vi "disdrometer_weathericon.vi"(0 "Weather Status":string, 5 "Time (seconds, GMT)":dbl, 7 "Offset (hours)":dbl, 9 "Begin Daylight (hours)":dbl=8.0, 11 "End Daylight (hours)":dbl=20.0) -> (6 "String":string, 10 "Icon":picture)   [LabVIEW 2018]
doc: "Accepts a SYNOP Tab.4680 weather code (e.g. \"R-\", \"R \", \"R+\", etc.) and returns a string description and the filepath to an associated icon.\n\nTime parameters can be optionally included to vary the icon based on a day/night cycle."
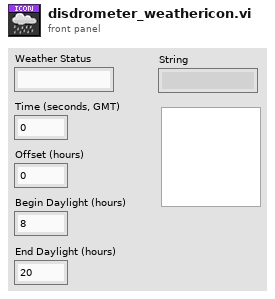
[diagram p1: front panel]
types:
  T1 = typedef "imagedata.ctl" = cluster{"image type":i32, "image depth":i32, "image":u8[], "mask":u8[], "colors":u32[], "Rectangle":cluster{"left":i16, "top":i16, "right":i16, "bottom":i16}}
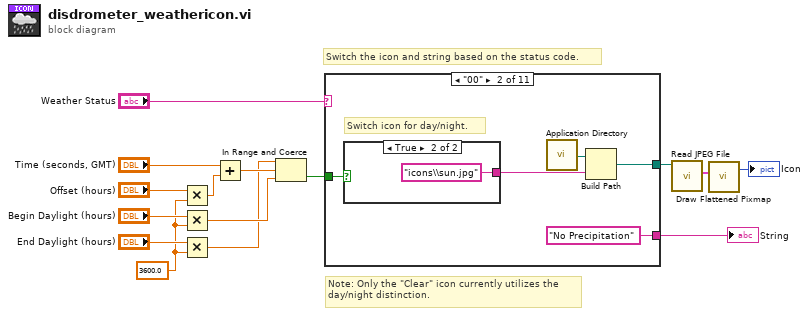
[diagram p0: block diagram]
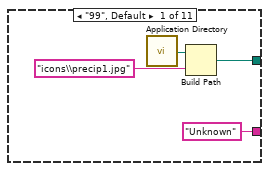
[diagram p2: hidden frame]
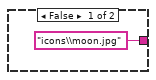
[diagram p3: hidden frame]
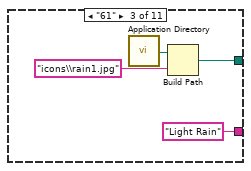
[diagram p4: hidden frame]
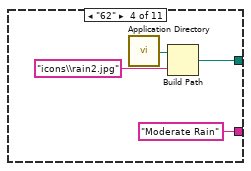
[diagram p5: hidden frame]
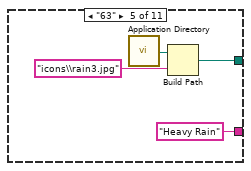
[diagram p6: hidden frame]
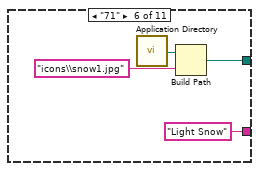
[diagram p7: hidden frame]
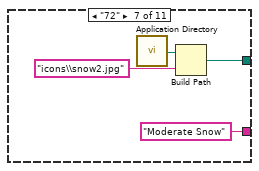
[diagram p8: hidden frame]
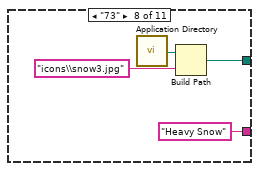
[diagram p9: hidden frame]
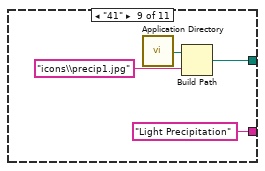
[diagram p10: hidden frame]
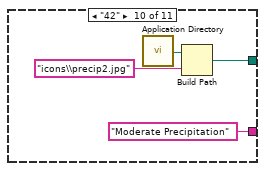
[diagram p11: hidden frame]
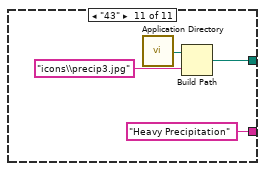
[diagram p12: hidden frame]
diagram:
  w6 = 3600.0 ("y")
  # "Switch the icon and string based on the status code."
  # "Note: Only the \"Clear\" icon currently utilizes the\nday/night distinction."
  n1 = Multiply(x="Offset (hours)", y=w6) -> (x*y=w10:dbl)
  n2 = Multiply(x="Begin Daylight (hours)", y=w6) -> (x*y=w5:dbl)
  n3 = Multiply(x="End Daylight (hours)", y=w6) -> (x*y=w4:dbl)
  n4 = Add(x="Time (seconds, GMT)", y=w10) -> (x+y=w8:dbl)
  n5 = In Range and Coerce(upper limit=w4, x=w8, lower limit=w5) -> (In Range?=w15:bool)  [unwired: 1 out]
  n6 = case shown="\"00\"" "Weather Status" {
    tunnel: ["Unknown" "No Precipitation" "Light Rain" "Moderate Rain" "Heavy Rain" "Light Snow" "Moderate Snow" "Heavy Snow" "Light Precipitation" "Moderate Precipitation" "Heavy Precipitation"] -> w13
    tunnel: [w16 w23 w27 w31 w35 w39 w43 w47 w51 w55 w59] -> w1
    tunnel: w15 -> [_ w21 _ _ _ _ _ _ _ _ _]
    frame "99", Default {
      n7 = call <vilib>:"Application Directory.vi"() -> ("Application Directory"=w18:path)
      n8 = Build Path(base path=w18, name or relative path="icons\\precip1.jpg") -> (appended path=w16:path)
    }
    frame "00" {
      # "Switch icon for day/night."
      n9 = case shown="True" w21 {
        tunnel: ["icons\\moon.jpg" "icons\\sun.jpg"] -> w20
        frame False {
        }
        frame True {
        }
      }
      n10 = call <vilib>:"Application Directory.vi"() -> ("Application Directory"=w22:path)
      n11 = Build Path(base path=w22, name or relative path=w20) -> (appended path=w23:path)
    }
    frame "61" {
      n12 = call <vilib>:"Application Directory.vi"() -> ("Application Directory"=w29:path)
      n13 = Build Path(base path=w29, name or relative path="icons\\rain1.jpg") -> (appended path=w27:path)
    }
    frame "62" {
      n14 = call <vilib>:"Application Directory.vi"() -> ("Application Directory"=w33:path)
      n15 = Build Path(base path=w33, name or relative path="icons\\rain2.jpg") -> (appended path=w31:path)
    }
    frame "63" {
      n16 = call <vilib>:"Application Directory.vi"() -> ("Application Directory"=w37:path)
      n17 = Build Path(base path=w37, name or relative path="icons\\rain3.jpg") -> (appended path=w35:path)
    }
    frame "71" {
      n18 = call <vilib>:"Application Directory.vi"() -> ("Application Directory"=w41:path)
      n19 = Build Path(base path=w41, name or relative path="icons\\snow1.jpg") -> (appended path=w39:path)
    }
    frame "72" {
      n20 = call <vilib>:"Application Directory.vi"() -> ("Application Directory"=w45:path)
      n21 = Build Path(base path=w45, name or relative path="icons\\snow2.jpg") -> (appended path=w43:path)
    }
    frame "73" {
      n22 = call <vilib>:"Application Directory.vi"() -> ("Application Directory"=w49:path)
      n23 = Build Path(base path=w49, name or relative path="icons\\snow3.jpg") -> (appended path=w47:path)
    }
    frame "41" {
      n24 = call <vilib>:"Application Directory.vi"() -> ("Application Directory"=w53:path)
      n25 = Build Path(base path=w53, name or relative path="icons\\precip1.jpg") -> (appended path=w51:path)
    }
    frame "42" {
      n26 = call <vilib>:"Application Directory.vi"() -> ("Application Directory"=w57:path)
      n27 = Build Path(base path=w57, name or relative path="icons\\precip2.jpg") -> (appended path=w55:path)
    }
    frame "43" {
      n28 = call <vilib>:"Application Directory.vi"() -> ("Application Directory"=w61:path)
      n29 = Build Path(base path=w61, name or relative path="icons\\precip3.jpg") -> (appended path=w59:path)
    }
  }
  "String" <- w13
  n30 = call <vilib>:"Read JPEG File.vi"("path to JPEG file"=w1) -> ("image data"=w3:T1)  [unwired: 8 in, 2 out]
  n31 = call <vilib>:"Draw Flattened Pixmap.vi"("image data"=w3) -> ("new picture"=→"Icon":picture)  [unwired: 8 in]
